vi "CRYSerial number headings.vi"(4 "header":enum16{"none", "standard", "custom"}(ring), 6 "Start of file":bool, 8 "Operator":bool, 9 "Comment":string, 10 "Include serial numbers (F)":bool, 11 "Table in":string[][](array[string])) -> (2 "Header out":string[][](array[string]), 3 "Table out":string[][](array[string]))   [LabVIEW 2013]
uses:
  Data/CRYData & result stacks global.vi
  CRYMainGlobal.vi
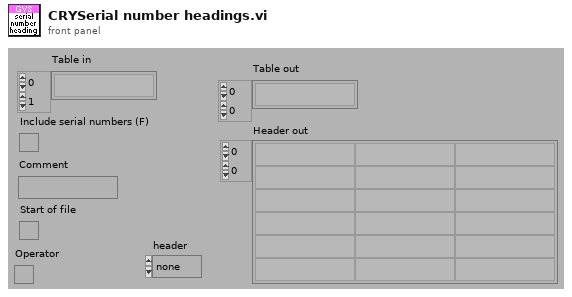
[diagram p1: front panel]
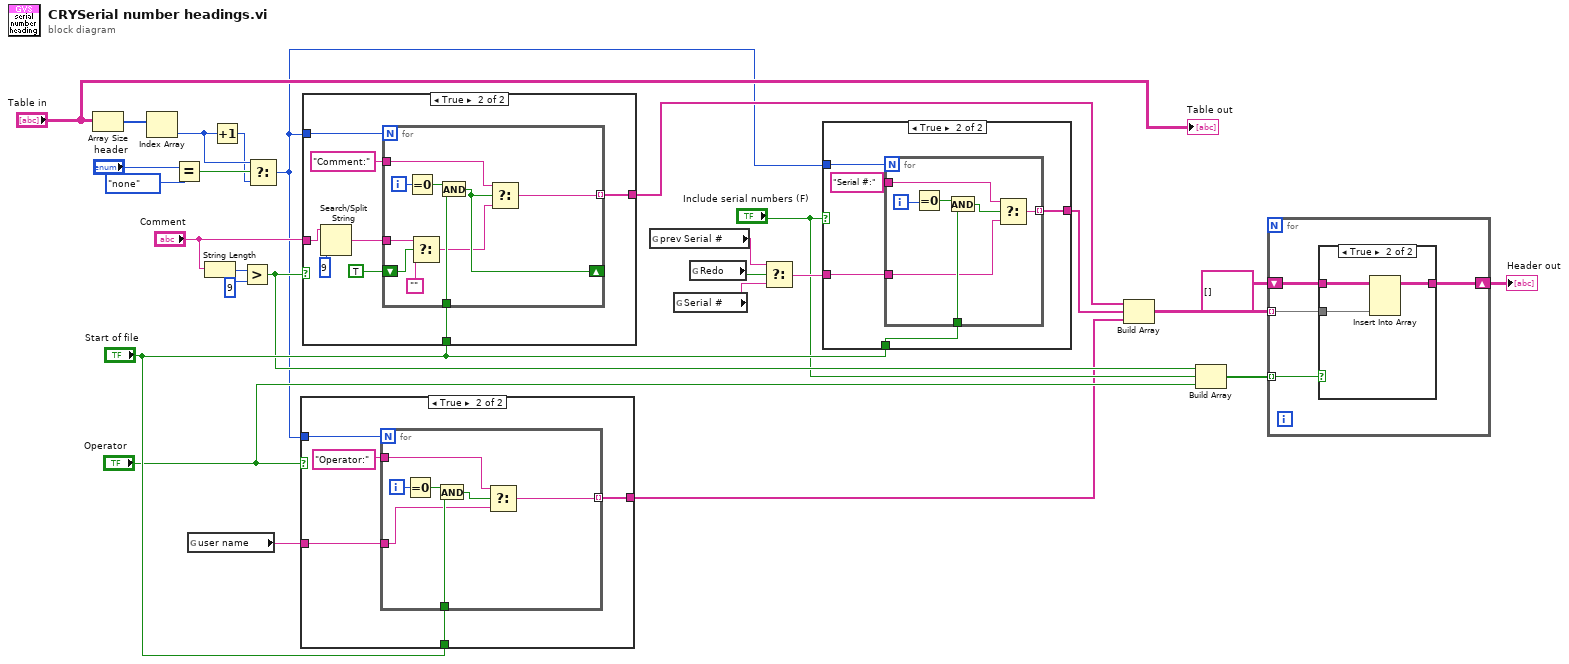
[diagram p0: block diagram]
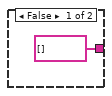
[diagram p3: hidden frame]
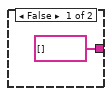
[diagram p4: hidden frame]
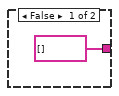
[diagram p5: hidden frame]
diagram:
  n1 = Array Size(array="Table in") -> (size(s)=w20:i32[])
  n2 = Index Array(array=w20) -> (element=w3:i32)  [unwired: 1 in]
  n3 = Equal?(x="header", y=enum16{"none", "standard", "custom"}."none") -> (x = y?=w6:bool)
  n4 = global read "CRYMainGlobal.vi" "user name"() -> (w16:string)
  n5 = String Length(string="Comment") -> (length=w26:i32)
  n6 = Increment(x=w3) -> (x+1=w2:i32)
  n7 = Greater?(x=w26, y=9) -> (0:w14:bool)
  n8 = Select(t=w3, s=w6, f=w2) -> (s? t:f=w1:i32)
  n9 = case shown="True" "Operator" {
    tunnel: "Start of file" -> [_ w33]
    tunnel: w1 -> [_ w31]
    tunnel: [string[] [] w32] -> w9
    tunnel: w16 -> [_ w30]
    frame False {
    }
    frame True {
      n10 = for {
        N: w31 -> [_]
        tunnel: w30 -> [w35]
        tunnel: w33 -> [w38]
        tunnel: [w36] -> w32 mode=indexing
        tunnel: "Operator:" -> [w34]
        i -> [w40]
        n11 = Equal To 0?(x=w40) -> (x = 0?=w39:bool)
        n12 = And(x=w39, y=w38) -> (x .and. y?=w37:bool)
        n13 = Select(t=w34, s=w37, f=w35) -> (s? t:f=w36:string)
      }
    }
  }
  n14 = case shown="True" w14 {
    tunnel: "Comment" -> [_ w48]
    tunnel: "Start of file" -> [_ w46]
    tunnel: w1 -> [_ w43]
    tunnel: [string[] [] w44] -> w18
    frame False {
    }
    frame True {
      n15 = Search/Split String(string=w48, offset (0)=9) -> (match + rest of string=w47:string)  [unwired: 3 out]
      n16 = for {
        N: w43 -> [_]
        tunnel: w47 -> [w55]
        tunnel: w46 -> [w57]
        shift-right: [w56] -> _
        shift-left: TRUE -> [w54]
        tunnel: [w51] -> w44 mode=indexing
        tunnel: "Comment:" -> [w50]
        i -> [w59]
        n17 = Equal To 0?(x=w59) -> (x = 0?=w58:bool)
        n18 = Select(t=w55, s=w54, f="") -> (s? t:f=w52:string)
        n19 = And(x=w58, y=w57) -> (x .and. y?=w56:bool)
        n20 = Select(t=w50, s=w56, f=w52) -> (s? t:f=w51:string)
      }
    }
  }
  n21 = global read "CRYData & result stacks global.vi" "prev Serial #"() -> (w22:string)
  n22 = global read "CRYData & result stacks global.vi" "Serial #"() -> (w21:string)
  n23 = global read "CRYData & result stacks global.vi" "Redo"() -> (w23:bool)
  n24 = Select(t=w22, s=w23, f=w21) -> (s? t:f=w24:string)
  n25 = case shown="True" "Include serial numbers (F)" {
    tunnel: [string[] [] w63] -> w10
    tunnel: w24 -> [_ w65]
    tunnel: "Start of file" -> [_ w64]
    tunnel: w1 -> [_ w62]
    frame False {
    }
    frame True {
      n26 = for {
        N: w62 -> [_]
        tunnel: w65 -> [w69]
        tunnel: w64 -> [w72]
        tunnel: [w67] -> w63 mode=indexing
        tunnel: "Serial #:" -> [w66]
        i -> [w71]
        n27 = Equal To 0?(x=w71) -> (x = 0?=w70:bool)
        n28 = And(x=w70, y=w72) -> (x .and. y?=w68:bool)
        n29 = Select(t=w66, s=w68, f=w69) -> (s? t:f=w67:string)
      }
    }
  }
  n30 = Build Array(w18, w10, w9) -> (w8:string[][])
  n31 = Build Array(w14, "Include serial numbers (F)", "Operator") -> (w11:bool[])
  n32 = for {
    shift-right: [w73] -> w7
    shift-left: string[][] [] -> [w76]
    tunnel: w11 -> [w75] mode=indexing
    tunnel: w8 -> [w74] mode=indexing
    n33 = case shown="True" w75 {
      tunnel: w76 -> [w77 w80]
      tunnel: w74 -> [_ w79]
      tunnel: [w77 w78] -> w73
      frame False {
      }
      frame True {
        n34 = Insert Into Array(array=w80, new element=w79) -> (w78:string[][])  [unwired: 2 in]
      }
    }
  }
  "Header out" <- w7
  "Table out" <- "Table in"
